vi "Read Fan Status.vi"(11 "更新风扇状态消息输入":refnum<class "Update Fan Status Msg.lvclass">) -> (1 "风扇B":T1, 2 "风扇A":T1)   [LabVIEW 2015, in "Dual Fan.lvlib" / "Update Fan Status Msg.lvclass"]
doc: "读取消息中记录的风扇状态。"
uses:
  Update Fan Status Msg.lvclass
  Dual Fan/Fan Info.ctl
  Update Fan Status Msg.lvclass/Update Fan Status Msg.ctl
  Dual Fan/Dual Fan.lvclass
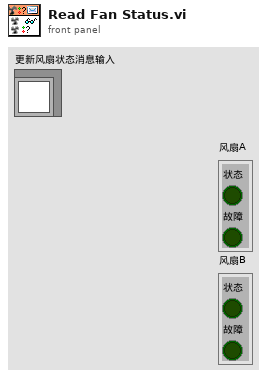
[diagram p1: front panel]
types:
  T1 = typedef "Dual Fan.lvlib/Dual Fan.lvclass/Fan Info.ctl" = cluster{"状态":bool, "故障":bool}
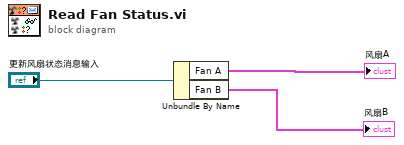
[diagram p0: block diagram]
diagram:
  n1 = Unbundle By Name("更新风扇状态消息输入") -> ("Fan A"=→"风扇A":T1, "Fan B"=→"风扇B":T1)
